vi "DI - PD500.vi"(8 "error in (no error)":errorcluster, 10 "Message IN":string) -> (0 "error out":errorcluster, 1 "Result (bool)":bool, 2 "Message OUT":string, 3 "VISA OUT":refnum<visa-resource-name>)   [LabVIEW 2022 SP3]
panel:
  out "Result (color)":u32(colorbox)
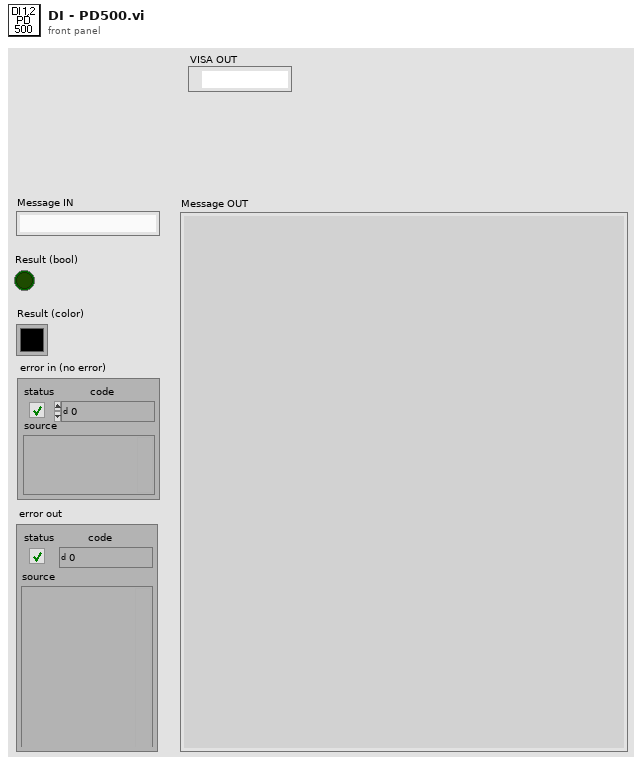
[diagram p1: front panel]
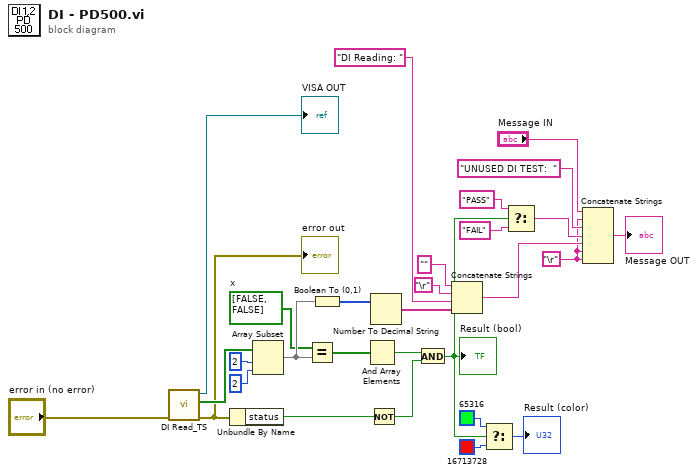
[diagram p0: block diagram]
diagram:
  w4 = bool[] [FALSE, FALSE]  # x
  w15 = "\r"
  n1 = call "DI Read_TS.vi"("error in (no error)"="error in (no error)") -> ("error out"=w1:errorcluster, "DI Reading"=w9:bool[], "VISA Refnum out"=→"VISA OUT":refnum<visa-resource-name>)  [unwired: 7 in, 1 out]
  "error out" <- w1
  n2 = Unbundle By Name(w1) -> ("status"=w24:bool)
  n3 = Array Subset(array=w9, index=2, length=2) -> (w5:bool[])
  n4 = Equal?(x=w4, y=w5) -> (x = y?=w6:bool[])
  n5 = Boolean To (0,1)(Boolean=w5) -> (0, 1=w12:i16[])
  n6 = And Array Elements(Boolean array=w6) -> (logical AND=w22:bool)
  n7 = Not(x=w24) -> (.not. x?=w21:bool)
  n8 = Number To Decimal String(number=w12) -> (decimal integer string=w7:string[])  [unwired: 1 in]
  n9 = And(x=w22, y=w21) -> (x .and. y?=w23:bool)
  "Result (bool)" <- w23
  n10 = Concatenate Strings("", "\r", "DI Reading: ", w7) -> (w20:string)
  n11 = Select(t=u32 65316 ("Result (color)"), s=w23, f=u32 16713728 ("Result (color)")) -> (s? t:f=→"Result (color)":u32)
  n12 = Select(t="PASS", s=w23, f="FAIL") -> (s? t:f=w17:string)
  n13 = Concatenate Strings("Message IN", w15, "UNUSED DI TEST:  ", w17, w20, w15, w15) -> (→"Message OUT":string)
